vi "ExAdvDispROI.vi"() -> ()   [LabVIEW 2010]
panel:
  in  "Clear ROI":bool
  in  "End ROI":bool
  in  "Start ROI":bool
  out "Y":u32
  out "X":u32
  out "Y":u32
  out "X":u32
  in  "Full File Name":path
  out "error out":errorcluster
  in  "error in (no error)":errorcluster
  in  "SITKFULLDISPLAYLib.SITKFullDisplay":refnum<k7>(container)
  # "Starting"
  # "Ending"
  # "Browse match pattern is set to *.tif.  Modify this if different file type is needed."
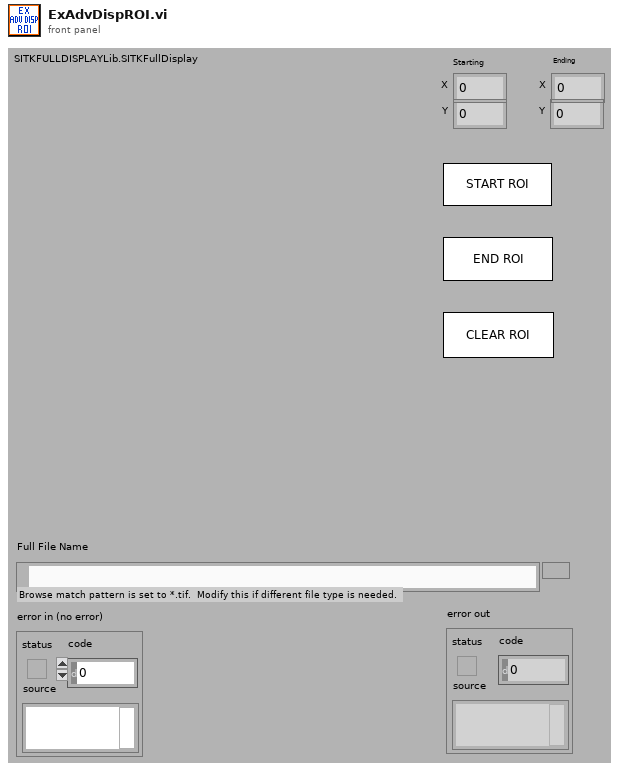
[diagram p1: front panel]
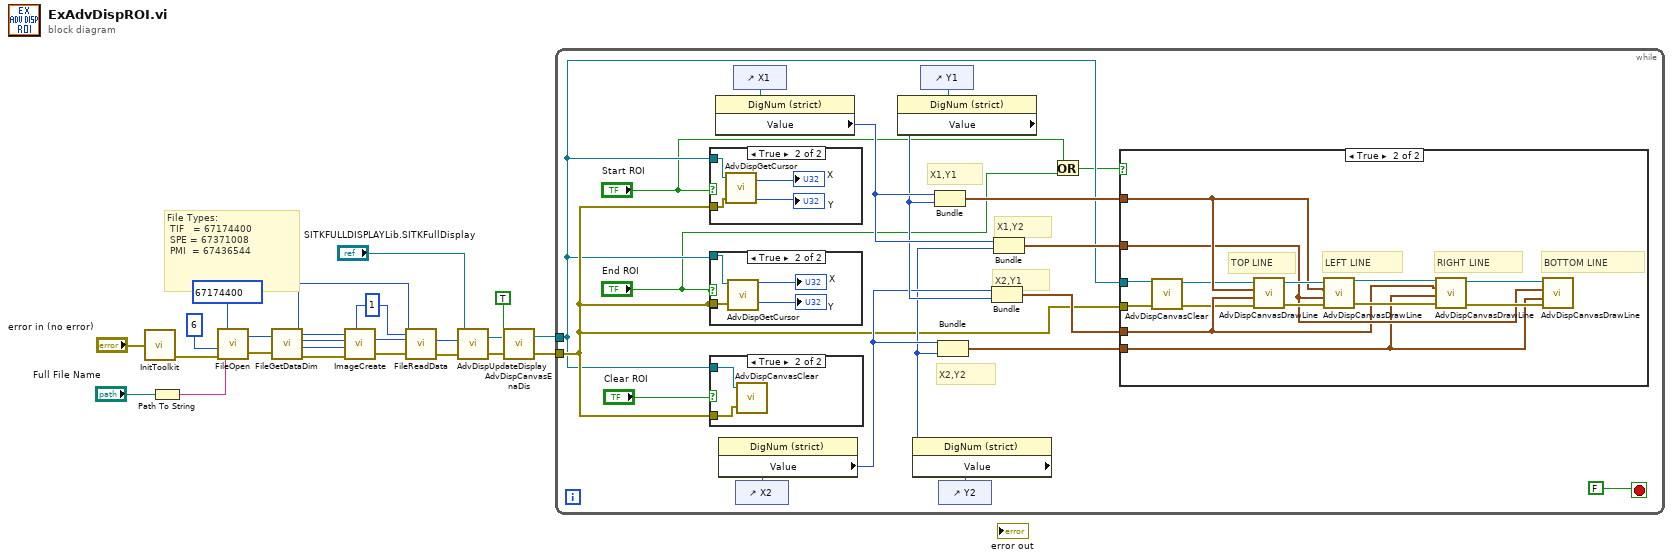
[diagram p0: block diagram]
diagram:
  w13 = 1
  # "File Types:\n TIF   = 67174400\n SPE = 67371008\n PMI  = 67436544"
  n1 = call <userlib>:"InitToolkit.vi"("error in"="error in (no error)") -> ("error out"=w9:errorcluster)
  n2 = Path To String(path="Full File Name") -> (string=w21:string)
  n3 = call <userlib>:"FileOpen.vi"("error in"=w9, "File Operations"=6, "FileName"=w21, "File Type"=67174400) -> ("error out"=w20:errorcluster, "File Handle"=w19:u32)
  n4 = call <userlib>:"FileGetDataDim.vi"("File Handle"=w19, "error in"=w20) -> ("Data Type"=w16:u32, "File Handle"=w14:u32, "X dim"=w18:u32, "Y dim"=w17:u32, "error out"=w15:errorcluster)  [unwired: 1 out]
  n5 = call <userlib>:"ImageCreate.vi"("X dimension"=w18, "Y dimension"=w17, "Data Type"=w16, "error in"=w15, "Number Of Frames"=w13) -> ("Image Handle"=w11:u32, "error out"=w12:errorcluster)
  n6 = call <userlib>:"FileReadData.vi"("File Handle"=w14, "Start Frame"=w13, "End Frame"=w13, "error in"=w12, "Image Handle"=w11) -> ("Image Handle"=w7:u32, "error out"=w6:errorcluster)  [unwired: 1 out]
  n7 = call <userlib>:"AdvDispUpdateDisplay.vi"("error in (no error)"=w6, "Image Handle"=w7, "SITKFULLDISPLAYLib.SITKFullDisplay"="SITKFULLDISPLAYLib.SITKFullDisplay") -> ("error out"=w3:errorcluster, "SITKFULLDISPLAYLib.SITKFullDisplay"=w4:refnum<k7>)  [unwired: 1 in]
  n8 = call <userlib>:"AdvDispCanvasEnaDis.vi"("error in (no error)"=w3, "Canvas enable"=TRUE, "SITKFULLDISPLAYLib.SITKFullDisplay"=w4) -> ("error out"=w2:errorcluster, "SITKFULLDISPLAYLib.SITKFullDisplay"=w1:refnum<k7>)
  n9 = while {
    tunnel: w2 -> [w29]
    tunnel: w1 -> [w28]
    stop <- FALSE stop-if-true
    # "X2,Y1"
    # "X1,Y2"
    # "X1,Y1"
    # "X2,Y2"
    n10 = case shown="True" "Start ROI" {
      tunnel: w29 -> [_ w67]
      tunnel: w28 -> [_ w66]
      frame False {
      }
      frame True {
        n11 = call <userlib>:"AdvDispGetCursor.vi"("SITKFULLDISPLAYLib.SITKFullDisplay"=w66, "error in (no error)"=w67) -> ("CursorX"=→"X":u32, "CursorY"=→"Y":u32)  [unwired: 2 out]
      }
    }
    n12 = case shown="True" "End ROI" {
      tunnel: w28 -> [_ w63]
      tunnel: w29 -> [_ _]
      tunnel: w29 -> [_ w62]
      frame False {
      }
      frame True {
        n13 = call <userlib>:"AdvDispGetCursor.vi"("SITKFULLDISPLAYLib.SITKFullDisplay"=w63, "error in (no error)"=w62) -> ("CursorX"=→"X":u32, "CursorY"=→"Y":u32)  [unwired: 2 out]
      }
    }
    n14 = case shown="True" "Clear ROI" {
      tunnel: w29 -> [_ w59]
      tunnel: w28 -> [_ w58]
      frame False {
      }
      frame True {
        n15 = call <userlib>:"AdvDispCanvasClear.vi"("error in (no error)"=w59, "SITKFULLDISPLAYLib.SITKFullDisplay"=w58) -> ()  [unwired: 2 out]
      }
    }
    n16 = control-ref of="X1"() -> (w38:refnum<vi>)
    n17 = property class="DigNum (strict)"(reference=w38) -> ("Value"=w37:u32)  [unwired: 1 in, 2 out]
    n18 = control-ref of="X2"() -> (w34:refnum<vi>)
    n19 = property class="DigNum (strict)"(reference=w34) -> ("Value"=w32:u32)  [unwired: 1 in, 2 out]
    n20 = control-ref of="Y1"() -> (w36:refnum<vi>)
    n21 = property class="DigNum (strict)"(reference=w36) -> ("Value"=w35:u32)  [unwired: 1 in, 2 out]
    n22 = Bundle("Value"=w37, "Value"=w35) -> (w42:cluster{"Value":u32, "Value":u32})  [unwired: 1 in]
    n23 = control-ref of="Y2"() -> (w33:refnum<vi>)
    n24 = property class="DigNum (strict)"(reference=w33) -> ("Value"=w31:u32)  [unwired: 1 in, 2 out]
    n25 = Bundle("Value"=w32, "Value"=w31) -> (w40:cluster{"Value":u32, "Value":u32})  [unwired: 1 in]
    n26 = Bundle("Value"=w32, "Value"=w35) -> (w30:cluster{"Value":u32, "Value":u32})  [unwired: 1 in]
    n27 = Bundle("Value"=w37, "Value"=w31) -> (w41:cluster{"Value":u32, "Value":u32})  [unwired: 1 in]
    n28 = Or(x="Start ROI", y="End ROI") -> (x .or. y?=w25:bool)
    n29 = case shown="True" w25 {
      tunnel: w42 -> [_ w55]
      tunnel: w41 -> [_ w50]
      tunnel: w40 -> [_ w49]
      tunnel: w30 -> [_ w48]
      tunnel: w29 -> [_ w44]
      tunnel: w28 -> [_ w47]
      frame False {
      }
      frame True {
        # "BOTTOM LINE"
        # "RIGHT LINE"
        # "LEFT LINE"
        # "TOP LINE"
        n30 = call <userlib>:"AdvDispCanvasClear.vi"("error in (no error)"=w44, "SITKFULLDISPLAYLib.SITKFullDisplay"=w47) -> ("error out"=w45:errorcluster, "SITKFULLDISPLAYLib.SITKFullDisplay"=w46:refnum<k7>)
        n31 = call <userlib>:"AdvDispCanvasDrawLine.vi"("error in (no error)"=w45, "Point 2"=w48, "Point 1"=w55, "SITKFULLDISPLAYLib.SITKFullDisplay"=w46) -> ("error out"=w56:errorcluster, "SITKFULLDISPLAYLib.SITKFullDisplay"=w57:refnum<k7>)
        n32 = call <userlib>:"AdvDispCanvasDrawLine.vi"("error in (no error)"=w56, "Point 2"=w50, "Point 1"=w55, "SITKFULLDISPLAYLib.SITKFullDisplay"=w57) -> ("error out"=w53:errorcluster, "SITKFULLDISPLAYLib.SITKFullDisplay"=w54:refnum<k7>)
        n33 = call <userlib>:"AdvDispCanvasDrawLine.vi"("error in (no error)"=w53, "Point 2"=w49, "Point 1"=w48, "SITKFULLDISPLAYLib.SITKFullDisplay"=w54) -> ("error out"=w51:errorcluster, "SITKFULLDISPLAYLib.SITKFullDisplay"=w52:refnum<k7>)
        n34 = call <userlib>:"AdvDispCanvasDrawLine.vi"("error in (no error)"=w51, "Point 2"=w49, "Point 1"=w50, "SITKFULLDISPLAYLib.SITKFullDisplay"=w52) -> ()  [unwired: 2 out]
      }
    }
  }
